vi "solar_type Script Type to Variant.vi"(6 "Array Delimiters (1D,2D)":string[](array[string]), 8 "error in (no error)":errorcluster, 9 "EnumItems":string[](array[string]), 10 "Value String":string, 11 "Type String":string) -> (0 "error out":errorcluster, 1 "Invalid?":bool, 2 "Value Variant":variant, 3 "Type":T1)   [LabVIEW 2018]
doc: "This converts the script type string to variant.\n\nTYPE = I8..I64,U8..U64,SGL,DBL,STR,BOOL,PATH,TIME\nTYPE_1D = 1D array (comma delimited)\nTYPE_2D = 2D array (comma & semicolon delimited)"
uses:
  <vilib>/Utility/Data Type/NI_Data Type.lvlib
  <vilib>/Utility/Data Type/Type Definitions/Memory Type.ctl
  <vilib>/Utility/Data Type/Type Definitions/Memory Info.ctl
  solar_type Item Type.ctl
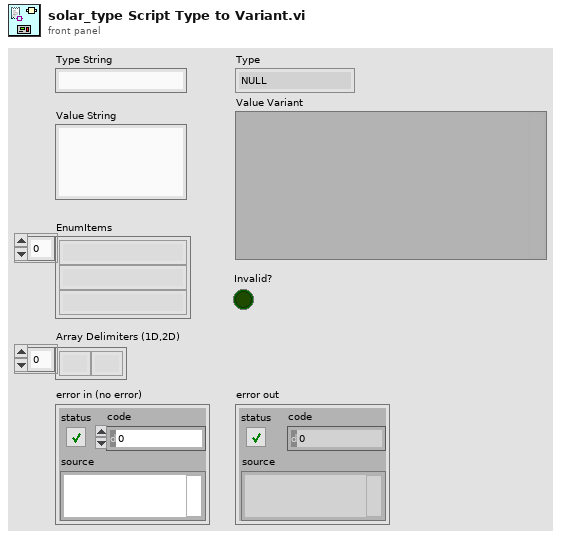
[diagram p1: front panel]
types:
  T1 = typedef "solar_type Item Type.ctl" = enum16{"NULL", "UNKNOWN", "CLUSTER", "I8", "I16", "I32", "I64", "U8", "U16", "U32", "U64", "U8_ENUM", "U16_ENUM", "U32_ENUM", "SGL", "DBL", "BOOLEAN", "STRING", "PATH", "VISA", "TAG", "TIME", "I8_1D", "I16_1D", "I32_1D", "I64_1D", "U8_1D", "U16_1D", "U32_1D", "U64_1D", "U8_ENUM_1D", "U16_ENUM_1D", "U32_ENUM_1D", "SGL_1D", "DBL_1D", "BOOLEAN_1D", "STRING_1D", "PATH_1D", "VISA_1D", "TAG_1D", "TIME_1D", "I8_2D", "I16_2D", "I32_2D", "I64_2D", "U8_2D", "U16_2D", "U32_2D", "U64_2D", "U8_ENUM_2D", "U16_ENUM_2D", "U32_ENUM_2D", "SGL_2D", "DBL_2D", "BOOLEAN_2D", "STRING_2D", "PATH_2D", "VISA_2D", "TAG_2D", "TIME_2D"}
  T2 = typedef "NI_Data Type.lvlib/Memory Info.ctl" = cluster{"Type":T3, "Size":u32}
  T3 = typedef "NI_Data Type.lvlib/Memory Type.ctl" = enum16{"Variable", "Fixed", "Bounded"}
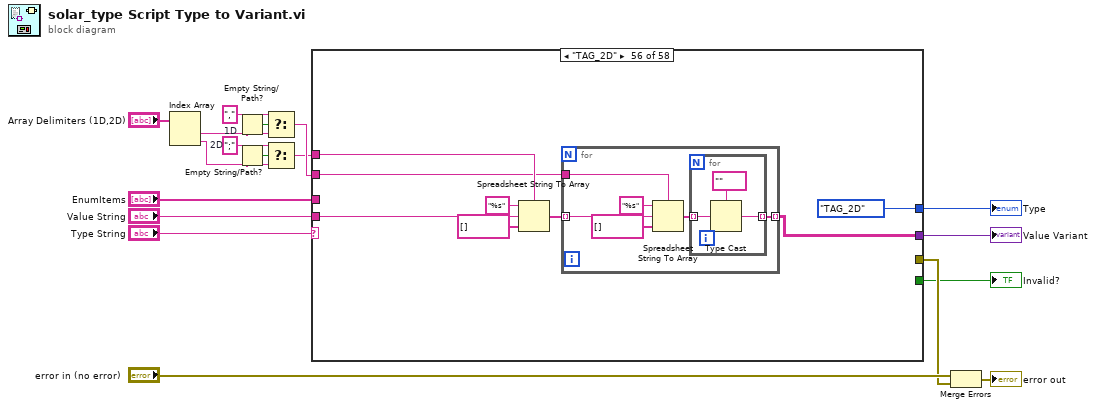
[diagram p0: block diagram]
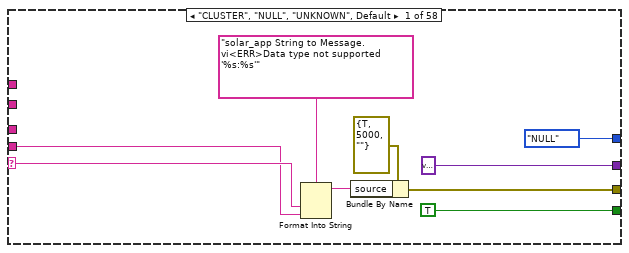
[diagram p2: hidden frame]
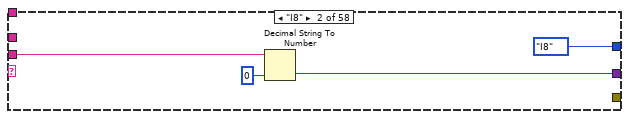
[diagram p3: hidden frame]
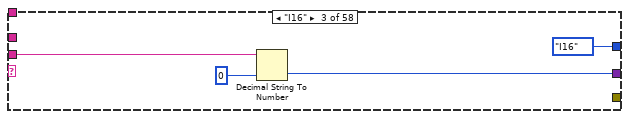
[diagram p4: hidden frame]
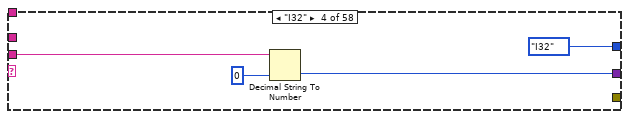
[diagram p5: hidden frame]
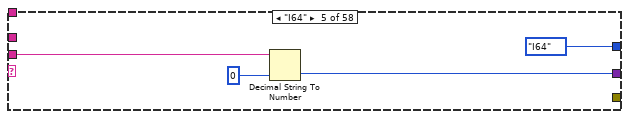
[diagram p6: hidden frame]
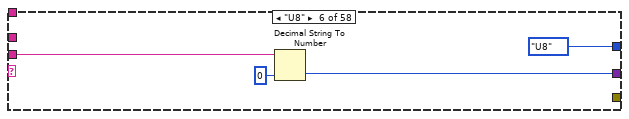
[diagram p7: hidden frame]
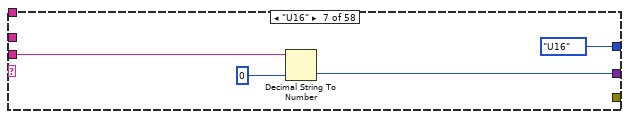
[diagram p8: hidden frame]
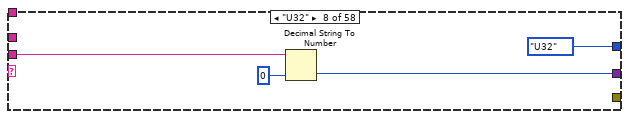
[diagram p9: hidden frame]
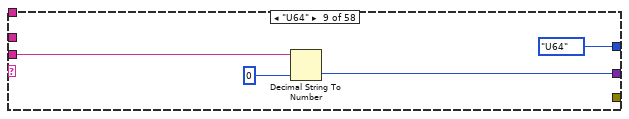
[diagram p10: hidden frame]
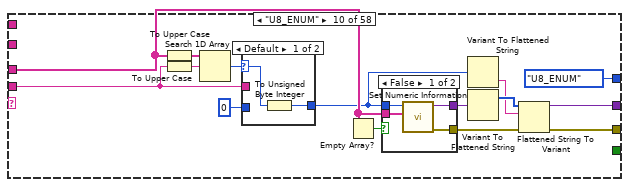
[diagram p11: hidden frame]
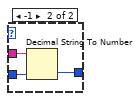
[diagram p12: hidden frame]
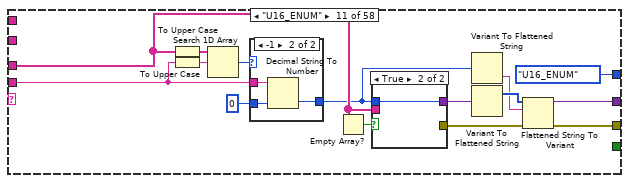
[diagram p14: hidden frame]
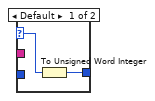
[diagram p15: hidden frame]
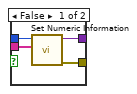
[diagram p16: hidden frame]
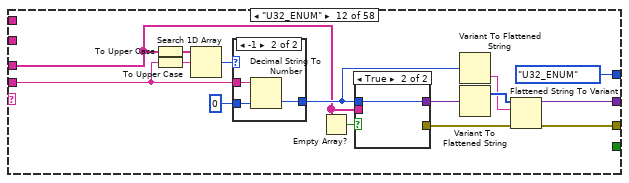
[diagram p17: hidden frame]
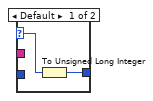
[diagram p18: hidden frame]
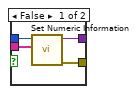
[diagram p19: hidden frame]
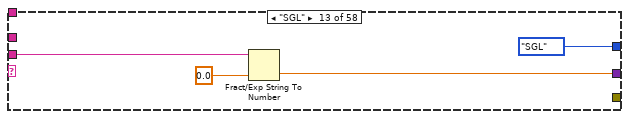
[diagram p20: hidden frame]
diagram:
  w4 = ";"  # 2D
  w6 = ","  # 1D
  n1 = Index Array(array="Array Delimiters (1D,2D)") -> (element #1=w7:string, element #2=w2:string)  [unwired: 2 in]
  n2 = Empty String/Path?(string/path=w7) -> (empty?=w8:bool)
  n3 = Empty String/Path?(string/path=w2) -> (empty?=w3:bool)
  n4 = Select(t=w6, s=w8, f=w7) -> (s? t:f=w5:string)
  n5 = Select(t=w4, s=w3, f=w2) -> (s? t:f=w1:string)
  n6 = case shown="\"TAG_2D\"" "Type String" {
    selector: "Type String" -> [w21 _ _ _ _ _ _ _ _ _ _ _ _ _ _ _ _ _ _ _ _ _ _ _ _ _ _ _ _ _ _ _ _ _ _ _ _ _ _ _ _ _ _ _ _ _ _ _ _ _ _ _ _ _ _ _ _ _]
    tunnel: [w24 _ _ _ _ _ _ _ _ w73 w95 w119 _ _ _ _ _ _ _ _ _ _ _ _ _ _ _ _ w229 w265 w301 _ _ _ _ _ _ _ _ _ _ _ _ _ _ _ _ w515 w560 w605 _ _ _ _ _ _ _ _] -> w12
    tunnel: [variant ("Variant") w29 w33 w37 w41 w45 w49 w53 w57 w68 w94 w118 w136 w140 w144 w149 w154 w158 w161 w165 w174 w180 w186 w192 w198 w204 w210 w216 w228 w264 w300 w331 w336 w342 w353 w358 w368 w379 w386 w401 w414 w427 w440 w453 w466 w479 w492 w514 w559 w604 w640 w653 w669 w687 w700 w717 w734 w748] -> w14
    tunnel: "EnumItems" -> [_ _ _ _ _ _ _ _ _ w63 w88 w115 _ _ _ _ _ _ _ _ _ _ _ _ _ _ _ _ w226 w262 w298 _ _ _ _ _ _ _ _ _ _ _ _ _ _ _ _ w512 w557 w602 _ _ _ _ _ _ _ _]
    tunnel: "Value String" -> [w20 w31 w35 w39 w43 w47 w51 w55 w59 w64 w89 w114 w138 w142 w145 w151 w155 w159 w162 w170 w178 w183 w189 w195 w201 w207 w213 w219 w234 w270 w306 w333 w339 w346 w356 w363 w373 w383 w389 w408 w421 w434 w447 w460 w473 w486 w499 w519 w564 w609 w647 w660 w672 w690 w703 w720 w737 w750]
    tunnel: [TRUE _ _ _ _ _ _ _ _ _ _ _ _ _ _ _ _ _ _ _ _ _ _ _ _ _ _ _ _ _ _ _ _ _ _ _ _ _ _ _ _ _ _ _ _ _ _ _ _ _ _ _ _ _ _ _ _ _] -> w10
    tunnel: w5 -> [_ _ _ _ _ _ _ _ _ _ _ _ _ _ _ _ _ _ _ _ w175 w182 w188 w194 w200 w206 w212 w218 w233 w269 w305 w330 w338 w344 w354 w361 w371 w381 w388 w402 w415 w428 w441 w454 w467 w480 w493 w506 w551 w596 w641 w654 w667 w685 w698 w715 w732 w746]
    tunnel: [solar_type_Item_Type."NULL" ("Type") solar_type_Item_Type."I8" ("Type") solar_type_Item_Type."I16" ("Type") solar_type_Item_Type."I32" ("Type") solar_type_Item_Type."I64" ("Type") solar_type_Item_Type."U8" ("Type") solar_type_Item_Type."U16" ("Type") solar_type_Item_Type."U32" ("Type") solar_type_Item_Type."U64" ("Type") solar_type_Item_Type."U8_ENUM" ("Type") solar_type_Item_Type."U16_ENUM" ("Type") solar_type_Item_Type."U32_ENUM" ("Type") solar_type_Item_Type."SGL" ("Type") solar_type_Item_Type."DBL" ("Type") solar_type_Item_Type."BOOLEAN" ("Type") solar_type_Item_Type."STRING" ("Type") solar_type_Item_Type."VISA" ("Type") solar_type_Item_Type."TAG" ("Type") solar_type_Item_Type."PATH" ("Type") solar_type_Item_Type."TIME" ("Type") solar_type_Item_Type."I8_1D" ("Type") solar_type_Item_Type."I16_1D" ("Type") solar_type_Item_Type."I32_1D" ("Type") solar_type_Item_Type."I64_1D" ("Type") solar_type_Item_Type."U8_1D" ("Type") solar_type_Item_Type."U16_1D" ("Type") solar_type_Item_Type."U32_1D" ("Type") solar_type_Item_Type."U64_1D" ("Type") solar_type_Item_Type."U8_ENUM_1D" ("Type") solar_type_Item_Type."U16_ENUM_1D" ("Type") solar_type_Item_Type."U32_ENUM_1D" ("Type") solar_type_Item_Type."SGL_1D" ("Type") solar_type_Item_Type."DBL_1D" ("Type") solar_type_Item_Type."BOOLEAN_1D" ("Type") solar_type_Item_Type."STRING_1D" ("Type") solar_type_Item_Type."VISA_1D" ("Type") solar_type_Item_Type."TAG_1D" ("Type") solar_type_Item_Type."PATH_1D" ("Type") solar_type_Item_Type."TIME_1D" ("Type") solar_type_Item_Type."I8_2D" ("Type") solar_type_Item_Type."I16_2D" ("Type") solar_type_Item_Type."I32_2D" ("Type") solar_type_Item_Type."I64_2D" ("Type") solar_type_Item_Type."U8_2D" ("Type") solar_type_Item_Type."U16_2D" ("Type") solar_type_Item_Type."U32_2D" ("Type") solar_type_Item_Type."U64_2D" ("Type") solar_type_Item_Type."U8_ENUM_2D" ("Type") solar_type_Item_Type."U16_ENUM_2D" ("Type") solar_type_Item_Type."U32_ENUM_2D" ("Type") solar_type_Item_Type."SGL_2D" ("Type") solar_type_Item_Type."DBL_2D" ("Type") solar_type_Item_Type."BOOLEAN_2D" ("Type") solar_type_Item_Type."STRING_2D" ("Type") solar_type_Item_Type."VISA_2D" ("Type") solar_type_Item_Type."TAG_2D" ("Type") solar_type_Item_Type."PATH_2D" ("Type") solar_type_Item_Type."TIME_2D" ("Type")] -> w15
    tunnel: w1 -> [_ _ _ _ _ _ _ _ _ _ _ _ _ _ _ _ _ _ _ _ _ _ _ _ _ _ _ _ _ _ _ _ _ _ _ _ _ _ _ w404 w417 w430 w443 w456 w469 w482 w495 w507 w552 w597 w643 w656 w668 w686 w699 w716 w733 w747]
    frame "CLUSTER", "NULL", "UNKNOWN", Default {
      n7 = Format Into String(format string="solar_app String to Message.vi<ERR>Data type not supported '%s:%s'" ("source"), w21, w20) -> (resulting string=w27:string)  [unwired: 2 in, 1 out]
      n8 = Bundle By Name(cluster=errorcluster {"status"=TRUE, "code"=5000, "source"=""} ("error out"), "source"=w27) -> (w24:errorcluster)
    }
    frame "I8" {
      n9 = Decimal String To Number(string=w31, default (0L)=i8 0) -> (number=w29:i8)  [unwired: 1 in, 1 out]
    }
    frame "I16" {
      n10 = Decimal String To Number(string=w35, default (0L)=i16 0) -> (number=w33:i16)  [unwired: 1 in, 1 out]
    }
    frame "I32" {
      n11 = Decimal String To Number(string=w39, default (0L)=0) -> (number=w37:i32)  [unwired: 1 in, 1 out]
    }
    frame "I64" {
      n12 = Decimal String To Number(string=w43, default (0L)=i64 0) -> (number=w41:i64)  [unwired: 1 in, 1 out]
    }
    frame "U8" {
      n13 = Decimal String To Number(string=w47, default (0L)=u8 0) -> (number=w45:u8)  [unwired: 1 in, 1 out]
    }
    frame "U16" {
      n14 = Decimal String To Number(string=w51, default (0L)=u16 0) -> (number=w49:u16)  [unwired: 1 in, 1 out]
    }
    frame "U32" {
      n15 = Decimal String To Number(string=w55, default (0L)=u32 0) -> (number=w53:u32)  [unwired: 1 in, 1 out]
    }
    frame "U64" {
      n16 = Decimal String To Number(string=w59, default (0L)=u64 0) -> (number=w57:u64)  [unwired: 1 in, 1 out]
    }
    frame "U8_ENUM" {
      n17 = To Upper Case(1:w63) -> (0:w67:string[])
      n18 = To Upper Case(1:w64) -> (0:w66:string)
      n19 = Search 1D Array(1D array=w67, element=w66) -> (index of element=w65:i32)  [unwired: 1 in]
      n20 = case shown="Default" w65 {
        selector: w65 -> [w76 _]
        tunnel: u8 0 -> [_ w79]
        tunnel: [w75 w78] -> w61
        tunnel: w64 -> [_ w77]
        frame Default {
          n21 = To Unsigned Byte Integer(number=w76) -> (unsigned 8bit integer=w75:u8)
        }
        frame -1 {
          n22 = Decimal String To Number(string=w77, default (0L)=w79) -> (number=w78:u8)  [unwired: 1 in, 1 out]
        }
      }
      n23 = Empty Array?(array=w63) -> (empty?=w74:bool)
      n24 = case shown="False" w74 {
        tunnel: w61 -> [w83 w84]
        tunnel: [w82 w84] -> w71
        tunnel: [w81 _] -> w72
        tunnel: w63 -> [w80 _]
        frame False {
          n25 = call <vilib>:"Set Numeric Information.vi"("Enum Names"=w80, "Variant in"=w83) -> ("error out"=w81:errorcluster, "Variant out"=w82:variant)  [unwired: 8 in]
        }
        frame True {
        }
      }
      n26 = Variant To Flattened String(Variant=w61) -> (data string=w69:string)  [unwired: 1 out]
      n27 = Variant To Flattened String(Variant=w71) -> (1:w70:i16[])  [unwired: 1 out]
      n28 = Flattened String To Variant(4:w72, 6:w69, 7:w70) -> (0:w73:errorcluster, 3:w68:variant)
    }
    frame "U16_ENUM" {
      n29 = To Upper Case(1:w88) -> (0:w92:string[])
      n30 = To Upper Case(1:w89) -> (0:w91:string)
      n31 = Search 1D Array(1D array=w92, element=w91) -> (index of element=w90:i32)  [unwired: 1 in]
      n32 = case shown="-1" w90 {
        selector: w90 -> [w101 _]
        tunnel: u16 0 -> [_ w104]
        tunnel: [w100 w103] -> w86
        tunnel: w89 -> [_ w102]
        frame Default {
          n33 = To Unsigned Word Integer(number=w101) -> (unsigned 16bit integer=w100:u16)
        }
        frame -1 {
          n34 = Decimal String To Number(string=w102, default (0L)=w104) -> (number=w103:u16)  [unwired: 1 in, 1 out]
        }
      }
      n35 = Empty Array?(array=w88) -> (empty?=w99:bool)
      n36 = case shown="True" w99 {
        tunnel: w86 -> [w108 w109]
        tunnel: [w107 w109] -> w93
        tunnel: [w106 _] -> w96
        tunnel: w88 -> [w105 _]
        frame False {
          n37 = call <vilib>:"Set Numeric Information.vi"("Enum Names"=w105, "Variant in"=w108) -> ("error out"=w106:errorcluster, "Variant out"=w107:variant)  [unwired: 8 in]
        }
        frame True {
        }
      }
      n38 = Variant To Flattened String(Variant=w86) -> (data string=w97:string)  [unwired: 1 out]
      n39 = Variant To Flattened String(Variant=w93) -> (1:w98:i16[])  [unwired: 1 out]
      n40 = Flattened String To Variant(4:w96, 6:w97, 7:w98) -> (0:w95:errorcluster, 3:w94:variant)
    }
    frame "U32_ENUM" {
      n41 = To Upper Case(1:w115) -> (0:w113:string[])
      n42 = To Upper Case(1:w114) -> (0:w112:string)
      n43 = Search 1D Array(1D array=w113, element=w112) -> (index of element=w111:i32)  [unwired: 1 in]
      n44 = case shown="-1" w111 {
        selector: w111 -> [w126 _]
        tunnel: u32 0 -> [_ w129]
        tunnel: [w125 w128] -> w116
        tunnel: w114 -> [_ w127]
        frame Default {
          n45 = To Unsigned Long Integer(number=w126) -> (unsigned 32bit integer=w125:u32)
        }
        frame -1 {
          n46 = Decimal String To Number(string=w127, default (0L)=w129) -> (number=w128:u32)  [unwired: 1 in, 1 out]
        }
      }
      n47 = Empty Array?(array=w115) -> (empty?=w124:bool)
      n48 = case shown="True" w124 {
        tunnel: w116 -> [w133 w134]
        tunnel: [w132 w134] -> w117
        tunnel: [w131 _] -> w120
        tunnel: w115 -> [w130 _]
        frame False {
          n49 = call <vilib>:"Set Numeric Information.vi"("Enum Names"=w130, "Variant in"=w133) -> ("error out"=w131:errorcluster, "Variant out"=w132:variant)  [unwired: 8 in]
        }
        frame True {
        }
      }
      n50 = Variant To Flattened String(Variant=w116) -> (data string=w121:string)  [unwired: 1 out]
      n51 = Variant To Flattened String(Variant=w117) -> (1:w122:i16[])  [unwired: 1 out]
      n52 = Flattened String To Variant(4:w120, 6:w121, 7:w122) -> (0:w119:errorcluster, 3:w118:variant)
    }
    frame "SGL" {
      n53 = Fract/Exp String To Number(string=w138, default (0 dbl)=sgl 0.0) -> (number=w136:sgl)  [unwired: 2 in, 1 out]
    }
    frame "DBL" {
      n54 = Fract/Exp String To Number(string=w142, default (0 dbl)=0.0) -> (number=w140:dbl)  [unwired: 2 in, 1 out]
    }
    frame "BOOL", "BOOLEAN" {
      n55 = case shown="\"1\", \"true\"" w145 {
        tunnel: [FALSE TRUE] -> w144
        frame Default {
        }
        frame "1", "true" {
        }
      }
    }
    frame "STR", "STRING" {
      # "remove label"
      n56 = Type Cast(type="", x=w151) -> (*(type *) &x=w149:string)
    }
    frame "VISA" {
      # "remove label"
      n57 = Type Cast(type=refnum<visa-resource-name> refnum, x=w155) -> (*(type *) &x=w154:refnum<visa-resource-name>)
    }
    frame "TAG" {
      # "remove label"
      n58 = Type Cast(type=tag "", x=w159) -> (*(type *) &x=w158:tag)
    }
    frame "PATH", "PTH" {
      n59 = String To Path(string=w162) -> (path=w161:path)
    }
    frame "TIME" {
      # "YYYY:MM:DD_hh:mm:ss.uuuuuu"
      n60 = Scan From String(format string="%<%Y-%#m-%#d_%#H:%#M:%#S>T", input string=w170, default 1=timestamp(0 s since 1904-01-01)) -> (remaining string=w168:string, output 1=w169:timestamp)  [unwired: 2 in, 2 out]
      n61 = Concatenate Strings("0" ("string"), w168) -> (w166:string)
      n62 = Fract/Exp String To Number(string=w166) -> (number=w164:dbl)  [unwired: 3 in, 1 out]
      n63 = Add(x=w169, y=w164) -> (x+y=w165:timestamp)
    }
    frame "I8_1D" {
      n64 = Spreadsheet String To Array(delimiter (Tab)=w175, format string="%d", spreadsheet string=w178, array type (2D Dbl)=i8[] []) -> (array=w174:i8[])
    }
    frame "I16_1D" {
      n65 = Spreadsheet String To Array(delimiter (Tab)=w182, format string="%d", spreadsheet string=w183, array type (2D Dbl)=i16[] []) -> (array=w180:i16[])
    }
    frame "I32_1D" {
      n66 = Spreadsheet String To Array(delimiter (Tab)=w188, format string="%d", spreadsheet string=w189, array type (2D Dbl)=i32[] []) -> (array=w186:i32[])
    }
    frame "I64_1D" {
      n67 = Spreadsheet String To Array(delimiter (Tab)=w194, format string="%d", spreadsheet string=w195, array type (2D Dbl)=i64[] []) -> (array=w192:i64[])
    }
    frame "U8_1D" {
      n68 = Spreadsheet String To Array(delimiter (Tab)=w200, format string="%d", spreadsheet string=w201, array type (2D Dbl)=u8[] []) -> (array=w198:u8[])
    }
    frame "U16_1D" {
      n69 = Spreadsheet String To Array(delimiter (Tab)=w206, format string="%d", spreadsheet string=w207, array type (2D Dbl)=u16[] []) -> (array=w204:u16[])
    }
    frame "U32_1D" {
      n70 = Spreadsheet String To Array(delimiter (Tab)=w212, format string="%d", spreadsheet string=w213, array type (2D Dbl)=u32[] []) -> (array=w210:u32[])
    }
    frame "U64_1D" {
      n71 = Spreadsheet String To Array(delimiter (Tab)=w218, format string="%d", spreadsheet string=w219, array type (2D Dbl)=u64[] []) -> (array=w216:u64[])
    }
    frame "U8_ENUM_1D" {
      w223 = u8 0
      n72 = Spreadsheet String To Array(delimiter (Tab)=w233, format string="%s", spreadsheet string=w234, array type (2D Dbl)=string[] []) -> (array=w224:string[])
      n73 = Empty Array?(array=w226) -> (empty?=w239:bool)
      n74 = for {
        tunnel: w226 -> [w243]
        tunnel: w224 -> [w242] mode=indexing
        tunnel: w223 -> [w241]
        tunnel: [w240] -> w222 mode=indexing
        n75 = To Upper Case(1:w243) -> (0:w246:string[])
        n76 = To Upper Case(1:w242) -> (0:w245:string)
        n77 = Search 1D Array(1D array=w246, element=w245) -> (index of element=w244:i32)  [unwired: 1 in]
        n78 = case shown="Default" w244 {
          selector: w244 -> [w248 _]
          tunnel: w241 -> [_ w251]
          tunnel: [w247 w250] -> w240
          tunnel: w242 -> [_ w249]
          frame Default {
            n79 = To Unsigned Byte Integer(number=w248) -> (unsigned 8bit integer=w247:u8)
          }
          frame -1 {
            n80 = Decimal String To Number(string=w249, default (0L)=w251) -> (number=w250:u8)  [unwired: 1 in, 1 out]
          }
        }
      }
      n81 = case shown="True" w239 {
        tunnel: w223 -> [w255 w256]
        tunnel: [w254 w256] -> w238
        tunnel: [w253 _] -> w236
        tunnel: w226 -> [w252 _]
        frame False {
          n82 = call <vilib>:"Set Numeric Information.vi"("Enum Names"=w252, "Variant in"=w255) -> ("error out"=w253:errorcluster, "Variant out"=w254:variant)  [unwired: 8 in]
        }
        frame True {
        }
      }
      n83 = call <vilib>:"Set Array Information.vi"("error in (no error)"=w236, "Array Lengths"=T2[] [{"Type"=enum."Variable", "Size"=0}], "Array Element"=w238, "Variant in"=w222) -> ("error out"=w230:errorcluster, "Variant out"=w227:variant)  [unwired: 6 in]
      n84 = Variant To Flattened String(Variant=w222) -> (data string=w231:string)  [unwired: 1 out]
      n85 = Variant To Flattened String(Variant=w227) -> (1:w232:i16[])  [unwired: 1 out]
      n86 = Flattened String To Variant(4:w230, 6:w231, 7:w232) -> (0:w229:errorcluster, 3:w228:variant)
    }
    frame "U16_ENUM_1D" {
      w259 = u16 0
      n87 = Spreadsheet String To Array(delimiter (Tab)=w269, format string="%s", spreadsheet string=w270, array type (2D Dbl)=string[] []) -> (array=w260:string[])
      n88 = Empty Array?(array=w262) -> (empty?=w275:bool)
      n89 = for {
        tunnel: w262 -> [w279]
        tunnel: w260 -> [w278] mode=indexing
        tunnel: w259 -> [w277]
        tunnel: [w276] -> w258 mode=indexing
        n90 = To Upper Case(1:w279) -> (0:w282:string[])
        n91 = To Upper Case(1:w278) -> (0:w281:string)
        n92 = Search 1D Array(1D array=w282, element=w281) -> (index of element=w280:i32)  [unwired: 1 in]
        n93 = case shown="Default" w280 {
          selector: w280 -> [w284 _]
          tunnel: w277 -> [_ w287]
          tunnel: [w283 w286] -> w276
          tunnel: w278 -> [_ w285]
          frame Default {
            n94 = To Unsigned Word Integer(number=w284) -> (unsigned 16bit integer=w283:u16)
          }
          frame -1 {
            n95 = Decimal String To Number(string=w285, default (0L)=w287) -> (number=w286:u16)  [unwired: 1 in, 1 out]
          }
        }
      }
      n96 = case shown="True" w275 {
        tunnel: w259 -> [w291 w292]
        tunnel: [w290 w292] -> w274
        tunnel: [w289 _] -> w272
        tunnel: w262 -> [w288 _]
        frame False {
          n97 = call <vilib>:"Set Numeric Information.vi"("Enum Names"=w288, "Variant in"=w291) -> ("error out"=w289:errorcluster, "Variant out"=w290:variant)  [unwired: 8 in]
        }
        frame True {
        }
      }
      n98 = call <vilib>:"Set Array Information.vi"("error in (no error)"=w272, "Array Lengths"=T2[] [{"Type"=enum."Variable", "Size"=0}], "Array Element"=w274, "Variant in"=w258) -> ("error out"=w266:errorcluster, "Variant out"=w263:variant)  [unwired: 6 in]
      n99 = Variant To Flattened String(Variant=w258) -> (data string=w267:string)  [unwired: 1 out]
      n100 = Variant To Flattened String(Variant=w263) -> (1:w268:i16[])  [unwired: 1 out]
      n101 = Flattened String To Variant(4:w266, 6:w267, 7:w268) -> (0:w265:errorcluster, 3:w264:variant)
    }
    frame "U32_ENUM_1D" {
      w295 = u32 0
      n102 = Spreadsheet String To Array(delimiter (Tab)=w305, format string="%s", spreadsheet string=w306, array type (2D Dbl)=string[] []) -> (array=w296:string[])
      n103 = Empty Array?(array=w298) -> (empty?=w311:bool)
      n104 = for {
        tunnel: w298 -> [w315]
        tunnel: w296 -> [w314] mode=indexing
        tunnel: w295 -> [w313]
        tunnel: [w312] -> w294 mode=indexing
        n105 = To Upper Case(1:w315) -> (0:w318:string[])
        n106 = To Upper Case(1:w314) -> (0:w317:string)
        n107 = Search 1D Array(1D array=w318, element=w317) -> (index of element=w316:i32)  [unwired: 1 in]
        n108 = case shown="Default" w316 {
          selector: w316 -> [w320 _]
          tunnel: w313 -> [_ w323]
          tunnel: [w319 w322] -> w312
          tunnel: w314 -> [_ w321]
          frame Default {
            n109 = To Unsigned Long Integer(number=w320) -> (unsigned 32bit integer=w319:u32)
          }
          frame -1 {
            n110 = Decimal String To Number(string=w321, default (0L)=w323) -> (number=w322:u32)  [unwired: 1 in, 1 out]
          }
        }
      }
      n111 = case shown="True" w311 {
        tunnel: w295 -> [w327 w328]
        tunnel: [w326 w328] -> w310
        tunnel: [w325 _] -> w308
        tunnel: w298 -> [w324 _]
        frame False {
          n112 = call <vilib>:"Set Numeric Information.vi"("Enum Names"=w324, "Variant in"=w327) -> ("error out"=w325:errorcluster, "Variant out"=w326:variant)  [unwired: 8 in]
        }
        frame True {
        }
      }
      n113 = call <vilib>:"Set Array Information.vi"("error in (no error)"=w308, "Array Lengths"=T2[] [{"Type"=enum."Variable", "Size"=0}], "Array Element"=w310, "Variant in"=w294) -> ("error out"=w302:errorcluster, "Variant out"=w299:variant)  [unwired: 6 in]
      n114 = Variant To Flattened String(Variant=w294) -> (data string=w303:string)  [unwired: 1 out]
      n115 = Variant To Flattened String(Variant=w299) -> (1:w304:i16[])  [unwired: 1 out]
      n116 = Flattened String To Variant(4:w302, 6:w303, 7:w304) -> (0:w301:errorcluster, 3:w300:variant)
    }
    frame "SGL_1D" {
      n117 = Spreadsheet String To Array(delimiter (Tab)=w330, format string="%e", spreadsheet string=w333, array type (2D Dbl)=sgl[] []) -> (array=w331:sgl[])
    }
    frame "DBL_1D" {
      n118 = Spreadsheet String To Array(delimiter (Tab)=w338, format string="%e", spreadsheet string=w339, array type (2D Dbl)=dbl[] []) -> (array=w336:dbl[])
    }
    frame "BOOL_1D", "BOOLEAN_1D" {
      n119 = Spreadsheet String To Array(delimiter (Tab)=w344, format string="%s", spreadsheet string=w346, array type (2D Dbl)=string[] []) -> (array=w343:string[])
      n120 = for {
        tunnel: w343 -> [w349] mode=indexing
        tunnel: [w348] -> w342 mode=indexing
        n121 = case shown="\"1\", \"true\"" w349 {
          tunnel: [FALSE TRUE] -> w348
          frame Default {
          }
          frame "1", "true" {
          }
        }
      }
    }
    frame "STR_1D", "STRING_1D" {
      n122 = Spreadsheet String To Array(delimiter (Tab)=w354, format string="%s", spreadsheet string=w356, array type (2D Dbl)=string[] []) -> (array=w353:string[])
    }
    frame "VISA_1D" {
      n123 = Spreadsheet String To Array(delimiter (Tab)=w361, format string="%s", spreadsheet string=w363, array type (2D Dbl)=string[] []) -> (array=w360:string[])
      n124 = for {
        tunnel: w360 -> [w367] mode=indexing
        tunnel: [w366] -> w358 mode=indexing
        n125 = Type Cast(type=refnum<visa-resource-name> refnum, x=w367) -> (*(type *) &x=w366:refnum<visa-resource-name>)
      }
    }
    frame "TAG_1D" {
      n126 = Spreadsheet String To Array(delimiter (Tab)=w371, format string="%s", spreadsheet string=w373, array type (2D Dbl)=string[] []) -> (array=w370:string[])
      n127 = for {
        tunnel: w370 -> [w377] mode=indexing
        tunnel: [w376] -> w368 mode=indexing
        n128 = Type Cast(type=tag "", x=w377) -> (*(type *) &x=w376:tag)
      }
    }
    frame "PATH_1D", "PTH_1D" {
      n129 = Spreadsheet String To Array(delimiter (Tab)=w381, format string="%s", spreadsheet string=w383, array type (2D Dbl)=string[] []) -> (array=w380:string[])
      n130 = String To Path(string=w380) -> (path=w379:path[])
    }
    frame "TIME_1D" {
      n131 = Spreadsheet String To Array(delimiter (Tab)=w388, format string="%s", spreadsheet string=w389, array type (2D Dbl)=string[] []) -> (array=w387:string[])
      n132 = for {
        tunnel: w387 -> [w393] mode=indexing
        tunnel: [w392] -> w386 mode=indexing
        # "YYYY:MM:DD_hh:mm:ss.uuuuuu"
        n133 = Scan From String(format string="%<%Y-%#m-%#d_%#H:%#M:%#S>T", input string=w393, default 1=timestamp(0 s since 1904-01-01)) -> (remaining string=w397:string, output 1=w398:timestamp)  [unwired: 2 in, 2 out]
        n134 = Concatenate Strings("0" ("string"), w397) -> (w395:string)
        n135 = Fract/Exp String To Number(string=w395) -> (number=w394:dbl)  [unwired: 3 in, 1 out]
        n136 = Add(x=w398, y=w394) -> (x+y=w392:timestamp)
      }
    }
    frame "I8_2D" {
      n137 = Spreadsheet String To Array(delimiter (Tab)=w404, format string="%s", spreadsheet string=w408, array type (2D Dbl)=string[] []) -> (array=w403:string[])
      n138 = for {
        tunnel: w403 -> [w411] mode=indexing
        tunnel: w402 -> [w410]
        tunnel: [w409] -> w401 mode=indexing
        n139 = Spreadsheet String To Array(delimiter (Tab)=w410, format string="%d", spreadsheet string=w411, array type (2D Dbl)=i8[] []) -> (array=w409:i8[])
      }
    }
    frame "I16_2D" {
      n140 = Spreadsheet String To Array(delimiter (Tab)=w417, format string="%s", spreadsheet string=w421, array type (2D Dbl)=string[] []) -> (array=w416:string[])
      n141 = for {
        tunnel: w416 -> [w424] mode=indexing
        tunnel: w415 -> [w423]
        tunnel: [w422] -> w414 mode=indexing
        n142 = Spreadsheet String To Array(delimiter (Tab)=w423, format string="%d", spreadsheet string=w424, array type (2D Dbl)=i16[] []) -> (array=w422:i16[])
      }
    }
    frame "I32_2D" {
      n143 = Spreadsheet String To Array(delimiter (Tab)=w430, format string="%s", spreadsheet string=w434, array type (2D Dbl)=string[] []) -> (array=w429:string[])
      n144 = for {
        tunnel: w429 -> [w437] mode=indexing
        tunnel: w428 -> [w436]
        tunnel: [w435] -> w427 mode=indexing
        n145 = Spreadsheet String To Array(delimiter (Tab)=w436, format string="%d", spreadsheet string=w437, array type (2D Dbl)=i32[] []) -> (array=w435:i32[])
      }
    }
    frame "I64_2D" {
      n146 = Spreadsheet String To Array(delimiter (Tab)=w443, format string="%s", spreadsheet string=w447, array type (2D Dbl)=string[] []) -> (array=w442:string[])
      n147 = for {
        tunnel: w442 -> [w450] mode=indexing
        tunnel: w441 -> [w449]
        tunnel: [w448] -> w440 mode=indexing
        n148 = Spreadsheet String To Array(delimiter (Tab)=w449, format string="%d", spreadsheet string=w450, array type (2D Dbl)=i64[] []) -> (array=w448:i64[])
      }
    }
    frame "U8_2D" {
      n149 = Spreadsheet String To Array(delimiter (Tab)=w456, format string="%s", spreadsheet string=w460, array type (2D Dbl)=string[] []) -> (array=w455:string[])
      n150 = for {
        tunnel: w455 -> [w463] mode=indexing
        tunnel: w454 -> [w462]
        tunnel: [w461] -> w453 mode=indexing
        n151 = Spreadsheet String To Array(delimiter (Tab)=w462, format string="%d", spreadsheet string=w463, array type (2D Dbl)=u8[] []) -> (array=w461:u8[])
      }
    }
    frame "U16_2D" {
      n152 = Spreadsheet String To Array(delimiter (Tab)=w469, format string="%s", spreadsheet string=w473, array type (2D Dbl)=string[] []) -> (array=w468:string[])
      n153 = for {
        tunnel: w468 -> [w476] mode=indexing
        tunnel: w467 -> [w475]
        tunnel: [w474] -> w466 mode=indexing
        n154 = Spreadsheet String To Array(delimiter (Tab)=w475, format string="%d", spreadsheet string=w476, array type (2D Dbl)=u16[] []) -> (array=w474:u16[])
      }
    }
    frame "U32_2D" {
      n155 = Spreadsheet String To Array(delimiter (Tab)=w482, format string="%s", spreadsheet string=w486, array type (2D Dbl)=string[] []) -> (array=w481:string[])
      n156 = for {
        tunnel: w481 -> [w489] mode=indexing
        tunnel: w480 -> [w488]
        tunnel: [w487] -> w479 mode=indexing
        n157 = Spreadsheet String To Array(delimiter (Tab)=w488, format string="%d", spreadsheet string=w489, array type (2D Dbl)=u32[] []) -> (array=w487:u32[])
      }
    }
    frame "U64_2D" {
      n158 = Spreadsheet String To Array(delimiter (Tab)=w495, format string="%s", spreadsheet string=w499, array type (2D Dbl)=string[] []) -> (array=w494:string[])
      n159 = for {
        tunnel: w494 -> [w502] mode=indexing
        tunnel: w493 -> [w501]
        tunnel: [w500] -> w492 mode=indexing
        n160 = Spreadsheet String To Array(delimiter (Tab)=w501, format string="%d", spreadsheet string=w502, array type (2D Dbl)=u64[] []) -> (array=w500:u64[])
      }
    }
    frame "U8_ENUM_2D" {
      w509 = u8 0
      n161 = Spreadsheet String To Array(delimiter (Tab)=w507, format string="%s", spreadsheet string=w519, array type (2D Dbl)=string[] []) -> (array=w510:string[])
      n162 = Empty Array?(array=w512) -> (empty?=w524:bool)
      n163 = for {
        tunnel: w512 -> [w532]
        tunnel: w510 -> [w527] mode=indexing
        tunnel: w509 -> [w531]
        tunnel: [w530] -> w508 mode=indexing
        tunnel: w506 -> [w525]
        n164 = Spreadsheet String To Array(delimiter (Tab)=w525, format string="%s", spreadsheet string=w527, array type (2D Dbl)=string[] []) -> (array=w526:string[])
        n165 = for {
          tunnel: w532 -> [w536]
          tunnel: w526 -> [w535] mode=indexing
          tunnel: w531 -> [w534]
          tunnel: [w533] -> w530 mode=indexing
          n166 = To Upper Case(1:w536) -> (0:w539:string[])
          n167 = To Upper Case(1:w535) -> (0:w538:string)
          n168 = Search 1D Array(1D array=w539, element=w538) -> (index of element=w537:i32)  [unwired: 1 in]
          n169 = case shown="-1" w537 {
            selector: w537 -> [w541 _]
            tunnel: w534 -> [_ w544]
            tunnel: [w540 w543] -> w533
            tunnel: w535 -> [_ w542]
            frame Default {
              n170 = To Unsigned Byte Integer(number=w541) -> (unsigned 8bit integer=w540:u8)
            }
            frame -1 {
              n171 = Decimal String To Number(string=w542, default (0L)=w544) -> (number=w543:u8)  [unwired: 1 in, 1 out]
            }
          }
        }
      }
      n172 = case shown="True" w524 {
        tunnel: w509 -> [w548 w549]
        tunnel: [w547 w549] -> w523
        tunnel: [w546 _] -> w521
        tunnel: w512 -> [w545 _]
        frame False {
          n173 = call <vilib>:"Set Numeric Information.vi"("Enum Names"=w545, "Variant in"=w548) -> ("error out"=w546:errorcluster, "Variant out"=w547:variant)  [unwired: 8 in]
        }
        frame True {
        }
      }
      n174 = call <vilib>:"Set Array Information.vi"("error in (no error)"=w521, "Array Lengths"=T2[] [{"Type"=enum."Variable", "Size"=0}, {"Type"=enum."Variable", "Size"=0}], "Array Element"=w523, "Variant in"=w508) -> ("error out"=w516:errorcluster, "Variant out"=w513:variant)  [unwired: 6 in]
      n175 = Variant To Flattened String(Variant=w508) -> (data string=w517:string)  [unwired: 1 out]
      n176 = Variant To Flattened String(Variant=w513) -> (1:w518:i16[])  [unwired: 1 out]
      n177 = Flattened String To Variant(4:w516, 6:w517, 7:w518) -> (0:w515:errorcluster, 3:w514:variant)
    }
    frame "U16_ENUM_2D" {
      w554 = u16 0
      n178 = Spreadsheet String To Array(delimiter (Tab)=w552, format string="%s", spreadsheet string=w564, array type (2D Dbl)=string[] []) -> (array=w555:string[])
      n179 = Empty Array?(array=w557) -> (empty?=w569:bool)
      n180 = for {
        tunnel: w557 -> [w577]
        tunnel: w555 -> [w572] mode=indexing
        tunnel: w554 -> [w576]
        tunnel: [w575] -> w553 mode=indexing
        tunnel: w551 -> [w570]
        n181 = Spreadsheet String To Array(delimiter (Tab)=w570, format string="%s", spreadsheet string=w572, array type (2D Dbl)=string[] []) -> (array=w571:string[])
        n182 = for {
          tunnel: w577 -> [w581]
          tunnel: w571 -> [w580] mode=indexing
          tunnel: w576 -> [w579]
          tunnel: [w578] -> w575 mode=indexing
          n183 = To Upper Case(1:w581) -> (0:w584:string[])
          n184 = To Upper Case(1:w580) -> (0:w583:string)
          n185 = Search 1D Array(1D array=w584, element=w583) -> (index of element=w582:i32)  [unwired: 1 in]
          n186 = case shown="-1" w582 {
            selector: w582 -> [w586 _]
            tunnel: w579 -> [_ w589]
            tunnel: [w585 w588] -> w578
            tunnel: w580 -> [_ w587]
            frame Default {
              n187 = To Unsigned Byte Integer(number=w586) -> (unsigned 8bit integer=w585:u8)
            }
            frame -1 {
              n188 = Decimal String To Number(string=w587, default (0L)=w589) -> (number=w588:u16)  [unwired: 1 in, 1 out]
            }
          }
        }
      }
      n189 = case shown="True" w569 {
        tunnel: w554 -> [w593 w594]
        tunnel: [w592 w594] -> w568
        tunnel: [w591 _] -> w566
        tunnel: w557 -> [w590 _]
        frame False {
          n190 = call <vilib>:"Set Numeric Information.vi"("Enum Names"=w590, "Variant in"=w593) -> ("error out"=w591:errorcluster, "Variant out"=w592:variant)  [unwired: 8 in]
        }
        frame True {
        }
      }
      n191 = call <vilib>:"Set Array Information.vi"("error in (no error)"=w566, "Array Lengths"=T2[] [{"Type"=enum."Variable", "Size"=0}, {"Type"=enum."Variable", "Size"=0}], "Array Element"=w568, "Variant in"=w553) -> ("error out"=w561:errorcluster, "Variant out"=w558:variant)  [unwired: 6 in]
      n192 = Variant To Flattened String(Variant=w553) -> (data string=w562:string)  [unwired: 1 out]
      n193 = Variant To Flattened String(Variant=w558) -> (1:w563:i16[])  [unwired: 1 out]
      n194 = Flattened String To Variant(4:w561, 6:w562, 7:w563) -> (0:w560:errorcluster, 3:w559:variant)
    }
    frame "U32_ENUM_2D" {
      w599 = u32 0
      n195 = Spreadsheet String To Array(delimiter (Tab)=w597, format string="%s", spreadsheet string=w609, array type (2D Dbl)=string[] []) -> (array=w600:string[])
      n196 = Empty Array?(array=w602) -> (empty?=w614:bool)
      n197 = for {
        tunnel: w602 -> [w622]
        tunnel: w600 -> [w617] mode=indexing
        tunnel: w599 -> [w621]
        tunnel: [w620] -> w598 mode=indexing
        tunnel: w596 -> [w615]
        n198 = Spreadsheet String To Array(delimiter (Tab)=w615, format string="%s", spreadsheet string=w617, array type (2D Dbl)=string[] []) -> (array=w616:string[])
        n199 = for {
          tunnel: w622 -> [w626]
          tunnel: w616 -> [w625] mode=indexing
          tunnel: w621 -> [w624]
          tunnel: [w623] -> w620 mode=indexing
          n200 = To Upper Case(1:w626) -> (0:w629:string[])
          n201 = To Upper Case(1:w625) -> (0:w628:string)
          n202 = Search 1D Array(1D array=w629, element=w628) -> (index of element=w627:i32)  [unwired: 1 in]
          n203 = case shown="-1" w627 {
            selector: w627 -> [w631 _]
            tunnel: w624 -> [_ w634]
            tunnel: [w630 w633] -> w623
            tunnel: w625 -> [_ w632]
            frame Default {
              n204 = To Unsigned Byte Integer(number=w631) -> (unsigned 8bit integer=w630:u8)
            }
            frame -1 {
              n205 = Decimal String To Number(string=w632, default (0L)=w634) -> (number=w633:u32)  [unwired: 1 in, 1 out]
            }
          }
        }
      }
      n206 = case shown="True" w614 {
        tunnel: w599 -> [w638 w639]
        tunnel: [w637 w639] -> w613
        tunnel: [w636 _] -> w611
        tunnel: w602 -> [w635 _]
        frame False {
          n207 = call <vilib>:"Set Numeric Information.vi"("Enum Names"=w635, "Variant in"=w638) -> ("error out"=w636:errorcluster, "Variant out"=w637:variant)  [unwired: 8 in]
        }
        frame True {
        }
      }
      n208 = call <vilib>:"Set Array Information.vi"("error in (no error)"=w611, "Array Lengths"=T2[] [{"Type"=enum."Variable", "Size"=0}, {"Type"=enum."Variable", "Size"=0}], "Array Element"=w613, "Variant in"=w598) -> ("error out"=w606:errorcluster, "Variant out"=w603:variant)  [unwired: 6 in]
      n209 = Variant To Flattened String(Variant=w598) -> (data string=w607:string)  [unwired: 1 out]
      n210 = Variant To Flattened String(Variant=w603) -> (1:w608:i16[])  [unwired: 1 out]
      n211 = Flattened String To Variant(4:w606, 6:w607, 7:w608) -> (0:w605:errorcluster, 3:w604:variant)
    }
    frame "SGL_2D" {
      n212 = Spreadsheet String To Array(delimiter (Tab)=w643, format string="%s", spreadsheet string=w647, array type (2D Dbl)=string[] []) -> (array=w642:string[])
      n213 = for {
        tunnel: w642 -> [w650] mode=indexing
        tunnel: w641 -> [w649]
        tunnel: [w648] -> w640 mode=indexing
        n214 = Spreadsheet String To Array(delimiter (Tab)=w649, format string="%e", spreadsheet string=w650, array type (2D Dbl)=sgl[] []) -> (array=w648:sgl[])
      }
    }
    frame "DBL_2D" {
      n215 = Spreadsheet String To Array(delimiter (Tab)=w656, format string="%s", spreadsheet string=w660, array type (2D Dbl)=string[] []) -> (array=w655:string[])
      n216 = for {
        tunnel: w655 -> [w663] mode=indexing
        tunnel: w654 -> [w662]
        tunnel: [w661] -> w653 mode=indexing
        n217 = Spreadsheet String To Array(delimiter (Tab)=w662, format string="%e", spreadsheet string=w663, array type (2D Dbl)=dbl[] []) -> (array=w661:dbl[])
      }
    }
    frame "BOOL_2D", "BOOLEAN_2D" {
      n218 = Spreadsheet String To Array(delimiter (Tab)=w668, format string="%s", spreadsheet string=w672, array type (2D Dbl)=string[] []) -> (array=w670:string[])
      n219 = for {
        tunnel: w670 -> [w676] mode=indexing
        tunnel: [w679] -> w669 mode=indexing
        tunnel: w667 -> [w674]
        n220 = Spreadsheet String To Array(delimiter (Tab)=w674, format string="%s", spreadsheet string=w676, array type (2D Dbl)=string[] []) -> (array=w675:string[])
        n221 = for {
          tunnel: w675 -> [w681] mode=indexing
          tunnel: [w680] -> w679 mode=indexing
          n222 = case shown="\"1\", \"true\"" w681 {
            tunnel: [FALSE TRUE] -> w680
            frame Default {
            }
            frame "1", "true" {
            }
          }
        }
      }
    }
    frame "STR_2D", "STRING_2D" {
      n223 = Spreadsheet String To Array(delimiter (Tab)=w686, format string="%s", spreadsheet string=w690, array type (2D Dbl)=string[] []) -> (array=w688:string[])
      n224 = for {
        tunnel: w688 -> [w694] mode=indexing
        tunnel: [w692] -> w687 mode=indexing
        tunnel: w685 -> [w693]
        n225 = Spreadsheet String To Array(delimiter (Tab)=w693, format string="%s", spreadsheet string=w694, array type (2D Dbl)=string[] []) -> (array=w692:string[])
      }
    }
    frame "VISA_2D" {
      n226 = Spreadsheet String To Array(delimiter (Tab)=w699, format string="%s", spreadsheet string=w703, array type (2D Dbl)=string[] []) -> (array=w701:string[])
      n227 = for {
        tunnel: w701 -> [w708] mode=indexing
        tunnel: [w705] -> w700 mode=indexing
        tunnel: w698 -> [w707]
        n228 = Spreadsheet String To Array(delimiter (Tab)=w707, format string="%s", spreadsheet string=w708, array type (2D Dbl)=string[] []) -> (array=w706:string[])
        n229 = for {
          tunnel: w706 -> [w713] mode=indexing
          tunnel: [w712] -> w705 mode=indexing
          n230 = Type Cast(type=refnum<visa-resource-name> refnum, x=w713) -> (*(type *) &x=w712:refnum<visa-resource-name>)
        }
      }
    }
    frame "TAG_2D" {
      n231 = Spreadsheet String To Array(delimiter (Tab)=w716, format string="%s", spreadsheet string=w720, array type (2D Dbl)=string[] []) -> (array=w718:string[])
      n232 = for {
        tunnel: w718 -> [w725] mode=indexing
        tunnel: [w722] -> w717 mode=indexing
        tunnel: w715 -> [w724]
        n233 = Spreadsheet String To Array(delimiter (Tab)=w724, format string="%s", spreadsheet string=w725, array type (2D Dbl)=string[] []) -> (array=w723:string[])
        n234 = for {
          tunnel: w723 -> [w730] mode=indexing
          tunnel: [w729] -> w722 mode=indexing
          n235 = Type Cast(type=tag "", x=w730) -> (*(type *) &x=w729:tag)
        }
      }
    }
    frame "PATH_2D", "PTH_2D" {
      n236 = Spreadsheet String To Array(delimiter (Tab)=w733, format string="%s", spreadsheet string=w737, array type (2D Dbl)=string[] []) -> (array=w735:string[])
      n237 = for {
        tunnel: w735 -> [w742] mode=indexing
        tunnel: [w739] -> w734 mode=indexing
        tunnel: w732 -> [w741]
        n238 = Spreadsheet String To Array(delimiter (Tab)=w741, format string="%s", spreadsheet string=w742, array type (2D Dbl)=string[] []) -> (array=w740:string[])
        n239 = String To Path(string=w740) -> (path=w739:path[])
      }
    }
    frame "TIME_2D" {
      n240 = Spreadsheet String To Array(delimiter (Tab)=w747, format string="%s", spreadsheet string=w750, array type (2D Dbl)=string[] []) -> (array=w749:string[])
      n241 = for {
        tunnel: w749 -> [w755] mode=indexing
        tunnel: [w758] -> w748 mode=indexing
        tunnel: w746 -> [w753]
        n242 = Spreadsheet String To Array(delimiter (Tab)=w753, format string="%s", spreadsheet string=w755, array type (2D Dbl)=string[] []) -> (array=w754:string[])
        n243 = for {
          tunnel: w754 -> [w760] mode=indexing
          tunnel: [w759] -> w758 mode=indexing
          # "YYYY:MM:DD_hh:mm:ss.uuuuuu"
          n244 = Scan From String(format string="%<%Y-%#m-%#d_%#H:%#M:%#S>T", input string=w760, default 1=timestamp(0 s since 1904-01-01)) -> (remaining string=w764:string, output 1=w765:timestamp)  [unwired: 2 in, 2 out]
          n245 = Concatenate Strings("0" ("string"), w764) -> (w762:string)
          n246 = Fract/Exp String To Number(string=w762) -> (number=w761:dbl)  [unwired: 3 in, 1 out]
          n247 = Add(x=w765, y=w761) -> (x+y=w759:timestamp)
        }
      }
    }
  }
  "Type" <- w15
  "Value Variant" <- w14
  "Invalid?" <- w10
  n248 = Merge Errors("error in (no error)", w12) -> (→"error out":errorcluster)
